vi "Write Vertical Scrollbar.vi"(10 "Vertical Scrollbar":bool, 11 "Flex Dialog in":refnum<class "Flex UI Dialog.lvclass">) -> (3 "Flex Dialog out":refnum<class "Flex UI Dialog.lvclass">)   [LabVIEW 2016, in "Flex UI Dialog.lvclass"]
uses:
  Flex UI Dialog.lvclass
  Flex UI Dialog.lvclass/Flex UI Dialog.ctl
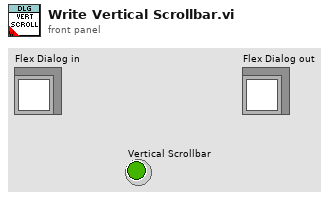
[diagram p1: front panel]
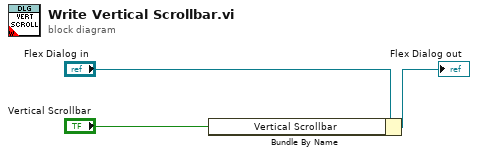
[diagram p0: block diagram]
diagram:
  n1 = Bundle By Name(cluster="Flex Dialog in", "Vertical Scrollbar"="Vertical Scrollbar") -> (→"Flex Dialog out":refnum<class "Flex UI Dialog.lvclass">)
